vi "VSI Scan Device.vi"(8 "error in (no error)":errorcluster, 11 "NeedInit":u8) -> (0 "error out":errorcluster, 3 "function return":i32)   [LabVIEW 2012, in "ControlSPI.lvlib"]
doc: "int WINAPI VSI_ScanDevice(unsigned char NeedInit=1);"
uses:
  ControlSPI.lvlib
  Ginkgo_Driver.dll
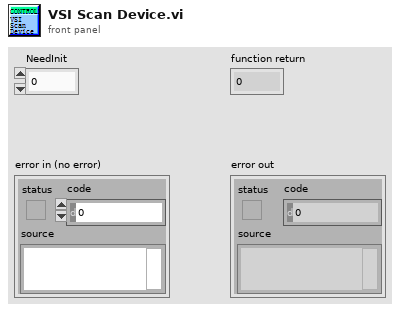
[diagram p1: front panel]
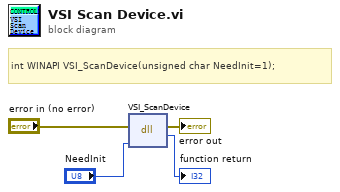
[diagram p0: block diagram]
diagram:
  # "int WINAPI VSI_ScanDevice(unsigned char NeedInit=1);"
  n1 = dll-call lib="E:/Project/vt_ginkgo/truck/Ginkgo Driver/vs2010/Ginkgo_USB-I2C_API_v2.0.3.0/lib/labview_32bit/ControlSPI/Ginkgo_Driver.*" fn="VSI_ScanDevice"(error in="error in (no error)", "NeedInit"="NeedInit") -> (error out=→"error out":errorcluster, →"function return":i32)  [unwired: 3 in, 1 out]
